vi "Initialize.vi"(8 "error in (no error)":errorcluster, 10 "Serial Configuration":T1={"Baud Rate"=9600, "Parity"=0, "Data Bits"=7, "Stop Bits"=10, "Flow Control"=0} {"Flow Control" items=["None", "XON/XOFF", "RTS/CTS", "XON/XOFF & RTS/CTS", "DTR/DSR", "XON/XOFF & DTR/DSR"]; "Stop Bits" items=["1.0"=10, "1.5"=15, "2.0"=20]; "Data Bits" items=["7"=7, "8"=8]; "Parity" items=["None", "Odd", "Even", "Mark", "Space"]; "Baud Rate" items=["300"=300, "600"=600, "1200"=1200, "2400"=2400, "4800"=4800, "9600"=9600, "19200"=19200, "115200"=115200]}, 11 "VISA resource name":refnum<visa-resource-name>) -> (0 "error out":errorcluster, 3 "VISA resource name out":refnum<visa-resource-name>)   [LabVIEW 2018, in "LTB-1.lvlib" / "3150.lvlib"]
doc: "Establishes communication with the instrument therefore, call this VI before calling other instrument driver VIs for this instrument. Generally, you need to call the <B>Initialize VI</B> only once at the beginning of an application."
uses:
  3150.lvlib
panel:
  # "(c) 2010 EXFO Inc. ALL RIGHTS RESERVED."
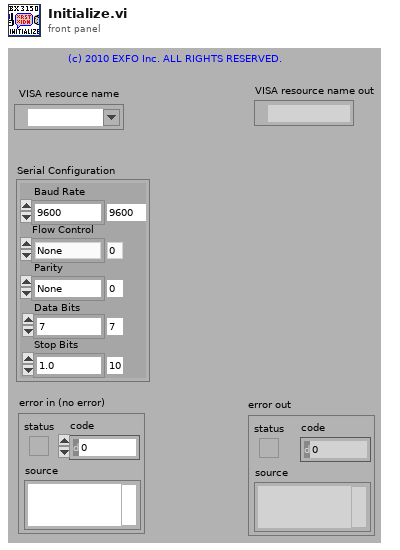
[diagram p1: front panel]
types:
  T1 = cluster{"Baud Rate":u32, "Parity":u16, "Data Bits":u16, "Stop Bits":u16, "Flow Control":u16}
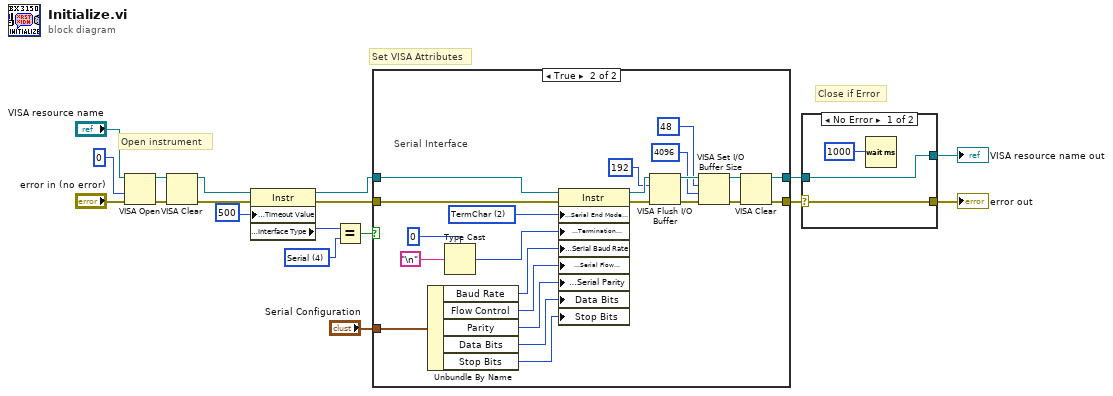
[diagram p0: block diagram]
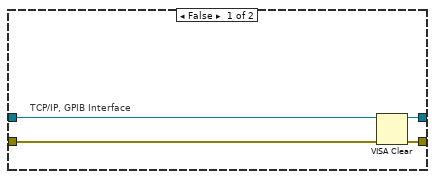
[diagram p2: hidden frame]
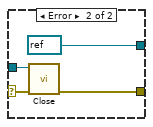
[diagram p3: hidden frame]
diagram:
  w8 = u16 4 items=["GPIB"=1, "VXI"=2, "GPIB-VXI"=3, "Serial"=4, "PXI"=5, "TCPIP"=6, "USB"=7] ("Interface Information:Interface Type")
  # "Set VISA Attributes"
  # "Close if Error"
  # "Open instrument"
  n1 = VISA Open(access mode=u32 0, error in (no error)="error in (no error)", VISA resource name="VISA resource name") -> (VISA resource name=w14:refnum<visa-resource-name>, error out=w13:errorcluster)  [unwired: 2 out]
  n2 = VISA Clear(VISA resource name=w14, error in (no error)=w13) -> (VISA resource name out=w12:refnum<visa-resource-name>, error out=w11:errorcluster)
  n3 = property class="Instr"(reference=w12, error in=w11, "General Settings:Timeout Value"=u32 500) -> (reference out=w17:refnum<visa-resource-name>, error out=w16:errorcluster, "Interface Information:Interface Type"=w7:u16)
  n4 = Equal?(x=w7, y=w8) -> (x = y?=w6:bool)
  n5 = case shown="True" w6 {
    tunnel: [w21 w24] -> w10
    tunnel: [w19 w23] -> w9
    tunnel: w17 -> [w22 w28]
    tunnel: w16 -> [w20 w27]
    tunnel: "Serial Configuration" -> [_ w31]
    frame False {
      # "TCP/IP, GPIB Interface"
      n6 = VISA Clear(VISA resource name=w22, error in (no error)=w20) -> (VISA resource name out=w21:refnum<visa-resource-name>, error out=w19:errorcluster)
    }
    frame True {
      w36 = u16 2 items=["None", "LastBit", "TermChar"] ("Serial Settings:Serial End Mode for Reads")
      # "Serial Interface"
      n7 = Unbundle By Name(w31) -> ("Baud Rate"=w34:u32, "Flow Control"=w32:u16, "Parity"=w33:u16, "Data Bits"=w29:u16, "Stop Bits"=w30:u16)
      n8 = Type Cast(type=u8 0, x="\n" ("Line Feed Constant")) -> (*(type *) &x=w35:u8)
      n9 = property class="Instr"(reference=w28, error in=w27, "Serial Settings:Serial End Mode for Reads"=w36, "Message Based Settings:Termination Character"=w35, "Serial Settings:Serial Baud Rate"=w34, "Serial Settings:Serial Flow Control"=w32, "Serial Settings:Serial Parity"=w33, "Data Bits"=w29, "Stop Bits"=w30) -> (reference out=w42:refnum<visa-resource-name>, error out=w44:errorcluster)
      n10 = VISA Flush I/O Buffer(VISA resource name=w42, mask (16)=u16 192, error in (no error)=w44) -> (VISA resource name out=w45:refnum<visa-resource-name>, error out=w43:errorcluster)
      n11 = VISA Set I/O Buffer Size(VISA resource name=w45, mask (16)=u16 48, size (4096)=u32 4096 ("size (0)"), error in (no error)=w43) -> (VISA resource name out=w26:refnum<visa-resource-name>, error out=w25:errorcluster)
      n12 = VISA Clear(VISA resource name=w26, error in (no error)=w25) -> (VISA resource name out=w24:refnum<visa-resource-name>, error out=w23:errorcluster)
    }
  }
  n13 = case shown="No Error" w9 {
    selector: w9 -> [w47 w49]
    tunnel: [w48 refnum<visa-resource-name> refnum ("VISA resource name out")] -> w5
    tunnel: [w47 w52] -> w2
    tunnel: w10 -> [w48 w50]
    frame No Error {
      n14 = Wait (ms)(milliseconds to wait=u32 1000) -> ()  [unwired: 1 out]
    }
    frame Error {
      n15 = call "Close.vi"("error in (no error)"=w49, "VISA resource name"=w50) -> ("error out"=w52:errorcluster)  [unwired: 9 out]
    }
  }
  "VISA resource name out" <- w5
  "error out" <- w2
